vi "enable disable stage controls.vi"(11 "Disabled":T1(ring)) -> ()   [LabVIEW 2012]
doc: "SciScan 1.2 160622"
uses:
  GFG/GFGfpRefGet.vi
  GFG/GFG library.lvlib
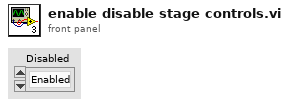
[diagram p1: front panel]
types:
  T1 = enum8{"Enabled", "Disabled", "Disabled and Grayed Out"}
  T2 = cluster{"WaveformChartRef":refnum<vi>, "DigitalRef":refnum<vi>, "ArrayRef":refnum<vi>, "TabControlRef":refnum<vi>, "EnumRef":refnum<vi>, "RingRef":refnum<vi>, "BooleanRef":refnum<vi>, "KnobRef":refnum<vi>, "SlideRef":refnum<vi>, "PathRef":refnum<vi>, "StringRef":refnum<vi>, "ComboBox":refnum<vi>, "WaveformGraphRef":refnum<vi>}
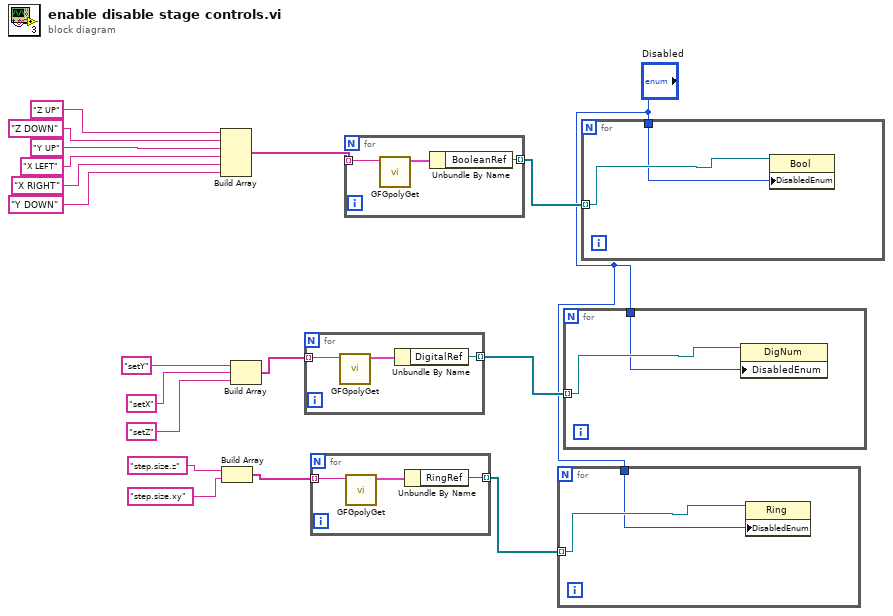
[diagram p0: block diagram]
diagram:
  n1 = Build Array("Z UP" ("Variable Name in"), "Z DOWN" ("Variable Name in"), "Y UP" ("Variable Name in"), "X LEFT" ("Variable Name in"), "X RIGHT" ("Variable Name in"), "Y DOWN" ("Variable Name in")) -> (w18:string[])
  n2 = Build Array("step.size.z", "step.size.xy") -> (w10:string[])
  n3 = Build Array("setY", "setX", "setZ") -> (w9:string[])
  n4 = for {
    tunnel: w9 -> [w20] mode=indexing
    tunnel: [w19] -> w3 mode=indexing
    n5 = call-poly "GFGpolyGet.vi"("Variable Name in"=w20) -> ("output cluster"=w21:T2)  [unwired: 9 in, 1 out]
    n6 = Unbundle By Name(w21) -> ("DigitalRef"=w19:refnum<vi>)
  }
  n7 = for {
    tunnel: w10 -> [w23] mode=indexing
    tunnel: [w22] -> w2 mode=indexing
    n8 = call-poly "GFGpolyGet.vi"("Variable Name in"=w23) -> ("output cluster"=w24:T2)  [unwired: 9 in, 1 out]
    n9 = Unbundle By Name(w24) -> ("RingRef"=w22:refnum<vi>)
  }
  n10 = for {
    tunnel: w18 -> [w26] mode=indexing
    tunnel: [w25] -> w11 mode=indexing
    n11 = call-poly "GFGpolyGet.vi"("Variable Name in"=w26) -> ("output cluster"=w27:T2)  [unwired: 9 in, 1 out]
    n12 = Unbundle By Name(w27) -> ("BooleanRef"=w25:refnum<vi>)
  }
  n13 = for {
    tunnel: w2 -> [w29] mode=indexing
    tunnel: "Disabled" -> [w28]
    n14 = property class="Ring"(reference=w29, "DisabledEnum"=w28) -> ()  [unwired: 1 in, 2 out]
  }
  n15 = for {
    tunnel: w3 -> [w31] mode=indexing
    tunnel: "Disabled" -> [w30]
    n16 = property class="DigNum"(reference=w31, "DisabledEnum"=w30) -> ()  [unwired: 1 in, 2 out]
  }
  n17 = for {
    tunnel: w11 -> [w33] mode=indexing
    tunnel: "Disabled" -> [w32]
    n18 = property class="Bool"(reference=w33, "DisabledEnum"=w32) -> ()  [unwired: 1 in, 2 out]
  }
